vi "SendMsg.vi"(8 "error in (no error)":errorcluster caption="错误输入（无错误）", 10 "Msg":string, 11 "Serve 输入":refnum<class "Serve.lvclass">) -> (0 "error out":errorcluster caption="错误输出", 3 "Serve 输出":refnum<class "Serve.lvclass">)   [LabVIEW 2024, in "Serve.lvlib" / "Serve.lvclass"]
uses:
  Serve.lvclass
  Serve.lvclass/Serve.ctl
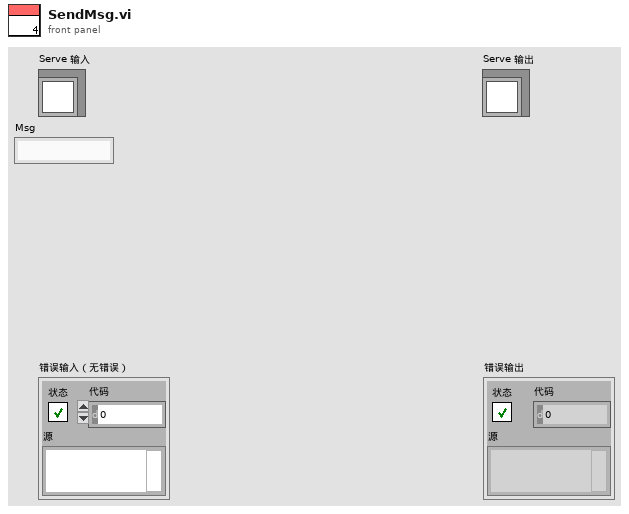
[diagram p1: front panel]
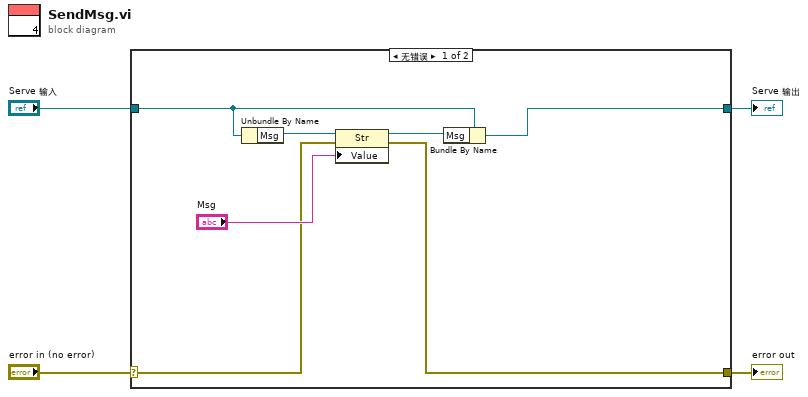
[diagram p0: block diagram]
diagram:
  n1 = case shown="无错误" "error in (no error)" {
    selector: "error in (no error)" -> [w6 w13]
    tunnel: [w5 w13] -> w3
    tunnel: [w7 w12] -> w1
    tunnel: "Serve 输入" -> [w9 w12]
    frame No Error {
      n2 = Unbundle By Name(w9) -> ("Msg"=w11:refnum<vi>)
      n3 = property class="Str"(reference=w11, error in=w6, "Value"="Msg") -> (reference out=w8:refnum<vi>, error out=w5:errorcluster)
      n4 = Bundle By Name(cluster=w9, "Msg"=w8) -> (w7:refnum<class "Serve.lvclass">)
    }
    frame Error {
    }
  }
  "error out" <- w3
  "Serve 输出" <- w1
